vi "Force fault trigger2.vi"(8 "error in (no error)":errorcluster, 10 "States.tau":dbl[](array[numeric]), 11 "Vessel in":refnum<class "Vessel.lvclass">) -> (0 "error out":errorcluster, 3 "Vessel out":refnum<class "Vessel.lvclass">)   [LabVIEW 2014, in "Vessel.lvclass"]
uses:
  Vessel.lvclass
  Vessel.lvclass/Vessel.ctl
panel:
  in  "Tab Control":enum32{"Page 1", "Page 2"}(tab)
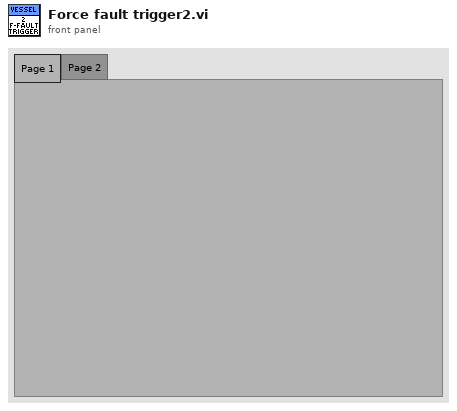
[diagram p1: front panel]
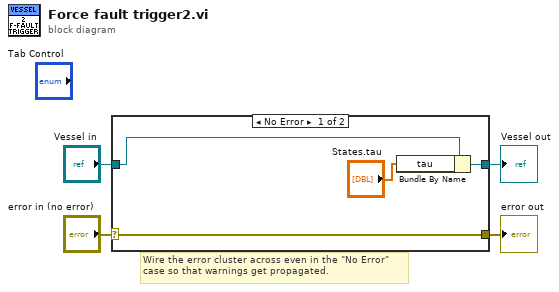
[diagram p0: block diagram]
diagram:
  # "Wire the error cluster across even in the \"No Error\"\ncase so that warnings get propagated."
  n1 = case shown="No Error" "error in (no error)" {
    selector: "error in (no error)" -> [w8 w10]
    tunnel: [w8 w10] -> w3
    tunnel: [w6 w9] -> w1
    tunnel: "Vessel in" -> [w7 w9]
    frame No Error {
      n2 = Bundle By Name(cluster=w7, "tau"="States.tau") -> (w6:refnum<class "Vessel.lvclass">)
    }
    frame Error {
    }
  }
  "error out" <- w3
  "Vessel out" <- w1
